vi "Untitled 1.vi"() -> (2 "distance":dbl)   [LabVIEW 2017]
uses:
  <vilib>/Rock Robotics/Network Tables/NT Read String.vi
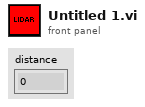
[diagram p1: front panel]
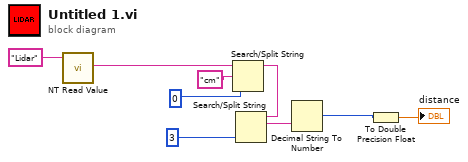
[diagram p0: block diagram]
diagram:
  n1 = call-poly <vilib>:"NT Read Value.vi"("Name"="Lidar") -> ("String"=w8:string)  [unwired: 9 in, 1 out]
  n2 = Search/Split String(string=w8, search string/char (-)="cm", offset (0)=0) -> (substring before match=w3:string)  [unwired: 2 out]
  n3 = Search/Split String(string=w3, offset (0)=3) -> (match + rest of string=w4:string)  [unwired: 1 in, 2 out]
  n4 = Decimal String To Number(string=w4) -> (number=w2:i32)  [unwired: 2 in, 1 out]
  n5 = To Double Precision Float(number=w2) -> (double precision float=→"distance":dbl)
